vi "record_sound.vi"(8 "error in (no error)":errorcluster, 10 "stop":bool, 11 "sound format":T1={"sample rate (S/s)"=22050.0, "number of channels"=2, "bits per sample"=16}) -> (0 "error out":errorcluster, 3 "data":waveform(dbl)[](array[waveform]))   [LabVIEW 2024]
uses:
  <vilib>/sound2/lvsound2.llb/Sound Data Format.ctl
  <vilib>/sound2/lvsound2.llb/Sampling Mode.ctl
  <vilib>/sound2/lvsound2.llb/Sound Input Read (DBL).vi
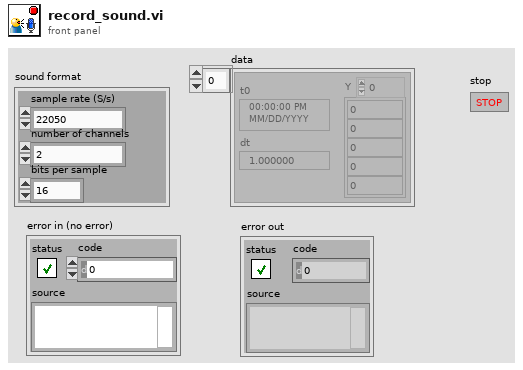
[diagram p1: front panel]
types:
  T1 = typedef "Sound Data Format.ctl" = cluster{"sample rate (S/s)":dbl, "number of channels":i32, "bits per sample":i32}
  T2 = typedef "Sampling Mode.ctl" = i32
  T3 = typedef "Sound Input Task ID.ctl" = u32
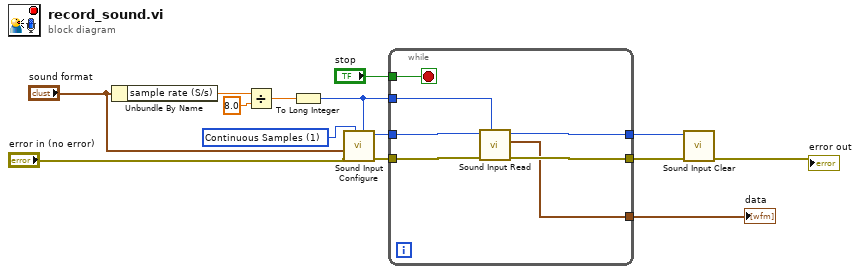
[diagram p0: block diagram]
diagram:
  w14 = T2 1 items=["Finite Samples", "Continuous Samples"] ("sample mode")
  n1 = Unbundle By Name("sound format") -> ("sample rate (S/s)"=w13:dbl)
  n2 = Divide(x=w13, y=8.0) -> (x/y=w11:dbl)
  n3 = To Long Integer(number=w11) -> (32bit integer=w5:i32)
  n4 = call <vilib>:"Sound Input Configure.vi"("number of samples/ch"=w5, "sample mode"=w14, "error in (no error)"="error in (no error)", "sound format"="sound format") -> ("error out"=w8:errorcluster, "task ID"=w10:T3)  [unwired: 6 in]
  n5 = while {
    tunnel: w10 -> [w21]
    tunnel: [w20] -> w9
    tunnel: w8 -> [w19]
    tunnel: [w18] -> w7
    tunnel: w5 -> [w17]
    tunnel: "stop" -> [w16]
    tunnel: [w15] -> w3
    stop <- w16 stop-if-true
    n6 = call-poly <vilib>:"Sound Input Read.vi"("number of samples/ch"=w17, "error in (no error)"=w19, "task ID"=w21) -> ("error out"=w18:errorcluster, "data"=w15:waveform(dbl)[], "task ID out"=w20:T3)  [unwired: 6 in]
  }
  "data" <- w3
  n7 = call <vilib>:"Sound Input Clear.vi"("error in (no error)"=w7, "task ID"=w9) -> ("error out"=→"error out":errorcluster)  [unwired: 9 in]
